vi "TwCloseAll.vi"(1 "error in (no error)":errorcluster) -> (0 "error out":errorcluster)   [LabVIEW 2009]
uses:
  TwH5Dll.dll
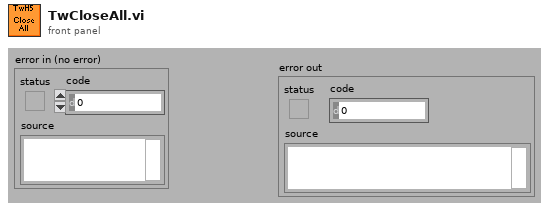
[diagram p1: front panel]
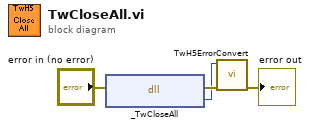
[diagram p0: block diagram]
diagram:
  n1 = dll-call lib="C:/src/85_TofDaq_current/DllWrappers/LabView/TwH5Dll/TwH5Dll.dll" fn="_TwCloseAll"(error in="error in (no error)") -> (error out=w3:errorcluster, "TwRetVal"=w2:i32)  [unwired: 2 in, 1 out]
  n2 = call "TwH5ErrorConvert.vi"("error in (no error)"=w3, "error code"=w2) -> ("error out"=→"error out":errorcluster)  [unwired: 9 out]
